vi "Prompt for Step.vi"(0 "Enable":bool=TRUE, 1 "Steps in":T2[](array[typedef]), 3 "Index In":i32=-1, 5 "error in (no error)":errorcluster) -> (16 "New Data Out":T2={"Type"=enum."Mouse Move", "Coords"={"x"=0, "y"=0}, "Delay"=0, "Key"=65, "Repeat"=0, "RClick?"=FALSE}, 18 "OK":bool, 19 "error out":errorcluster)   [LabVIEW 2021]
doc: "Prompts to enter a new step in the profile."
uses:
  CTLs/Step.ctl
  CTLs/Step Type.ctl
  <vilib>/Utility/inputDevices.llb/mouseAcquire.vi
  <vilib>/Utility/inputDevices.llb/closeMouse.vi
panel:
  in  "Repeat Amount":i32 min=0
  in  "Tab Control":enum32{"Coords", "RClick", "Key", "Nothing"}(tab)
  in  "Coords":cluster{"horizontal":i32, "vertical":i32}
  in  "Right Click?":bool
  in  "Key":u8(ring)=65
  in  "Delay (ms)":i32=100 min=0
  out "Step Type Description":string
  in  "Step Type":T1
  in  "Cancel":bool
  in  "OK":bool caption="OK2"
  # "Left and right click at\nsame time to capture\ncurrent screen coords"
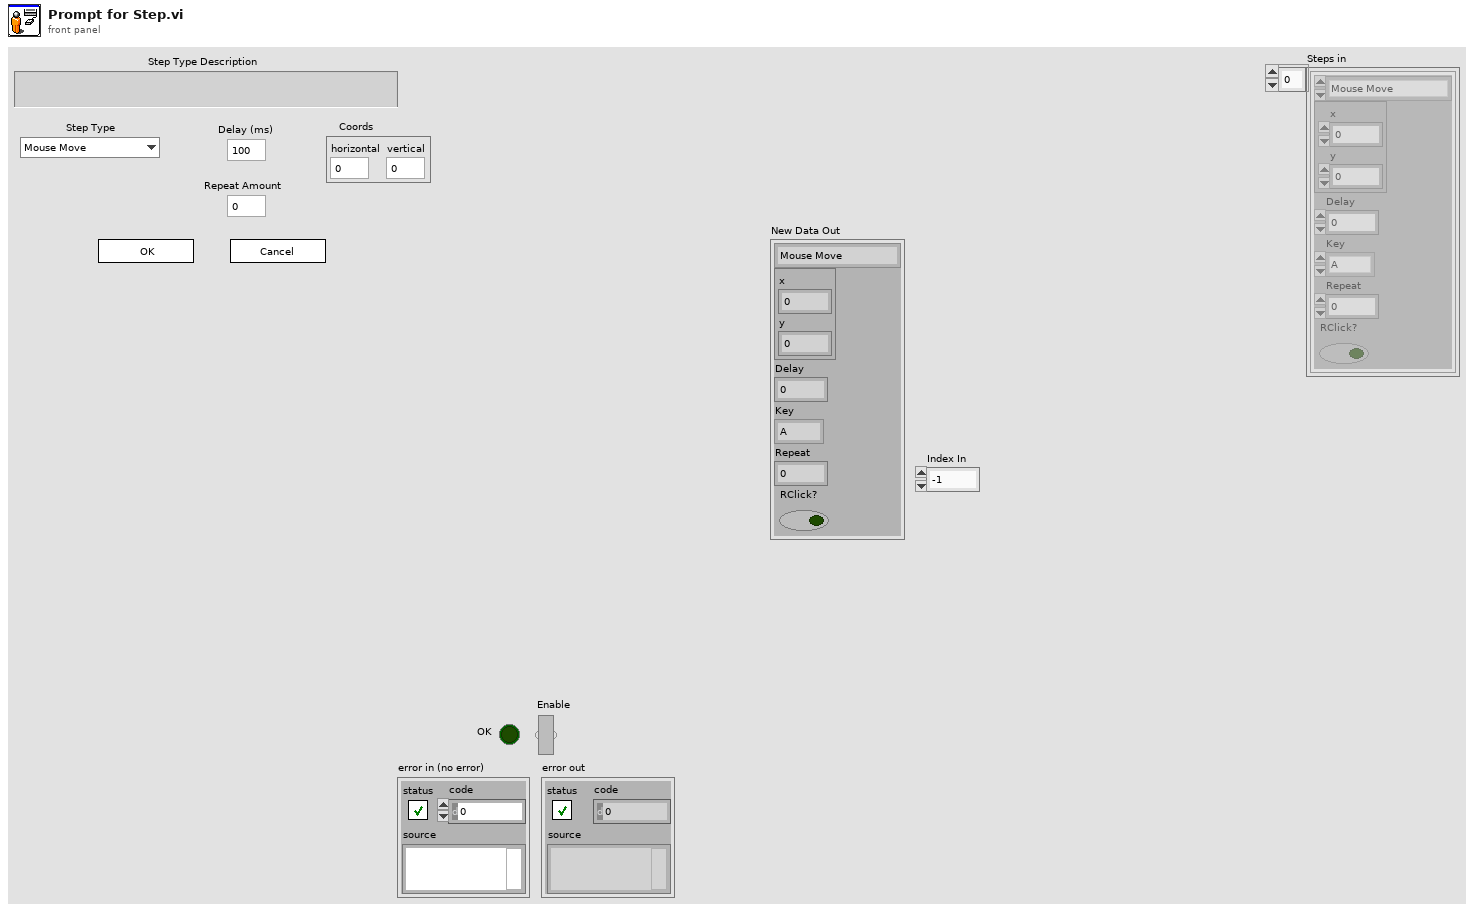
[diagram p1: front panel]
types:
  T1 = typedef "Step Type.ctl" = enum16{"Mouse Move", "Mouse Click", "Key Press", "Wait", "Mouse Down", "Mouse Up", "Key Down", "Key Up"}
  T2 = typedef "Step.ctl" = cluster{"Type":T1, "Coords":cluster{"x":i32, "y":i32}, "Delay":i32, "Key":u8, "Repeat":i32, "RClick?":bool}
  T3 = cluster{"Horizontal":i32, "Vertical":i32, "Scrolling":i32}
  T4 = cluster{"button 1":bool, "button 2":bool, "button 3":bool, "button 4":bool}
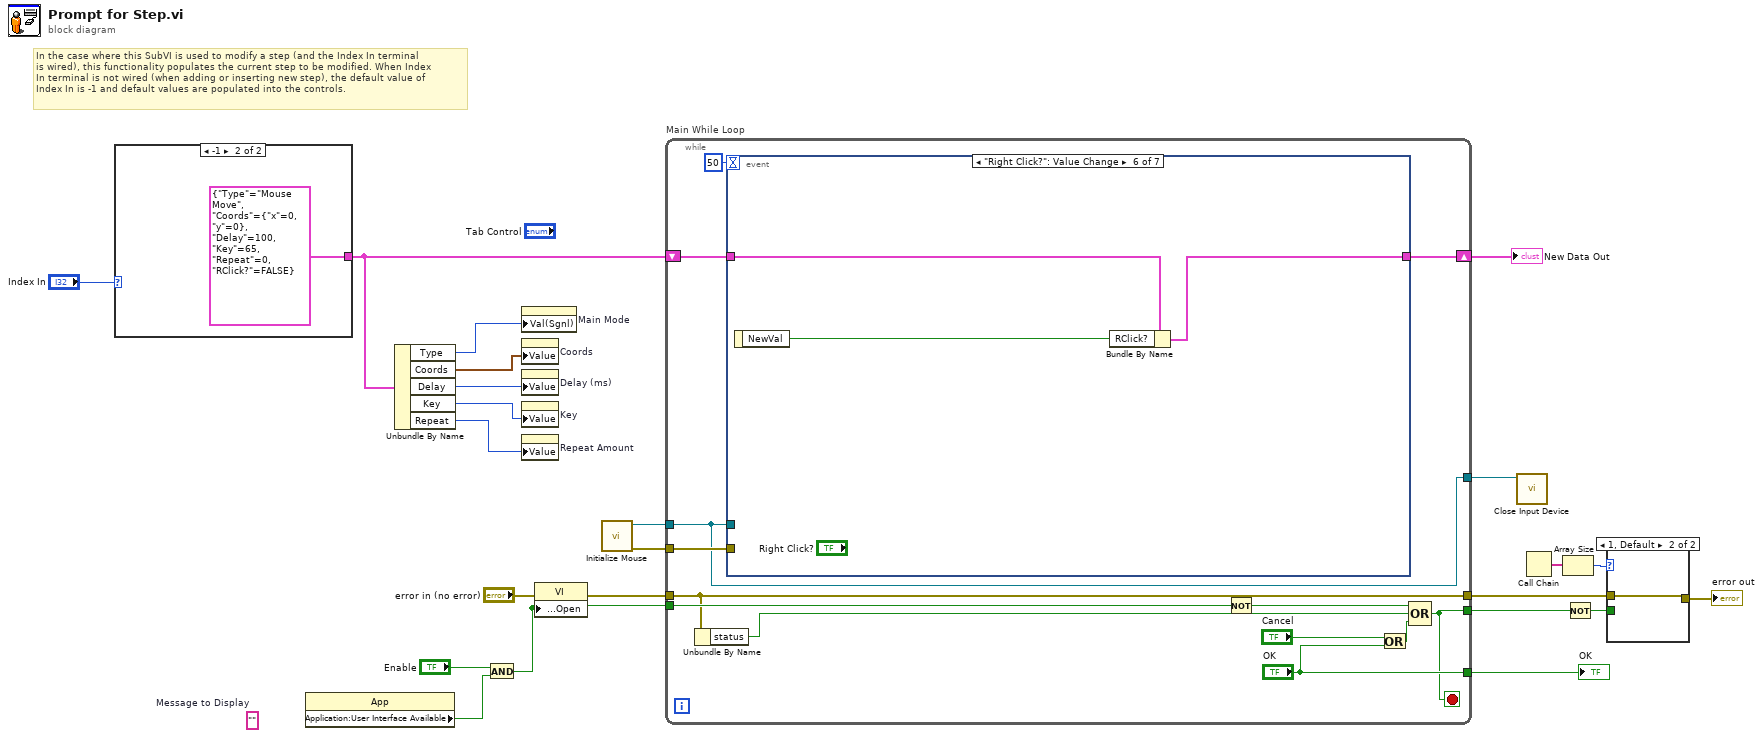
[diagram p0: block diagram]
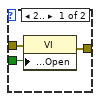
[diagram p2: hidden frame]
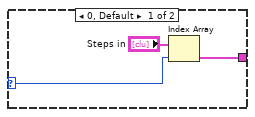
[diagram p3: hidden frame]
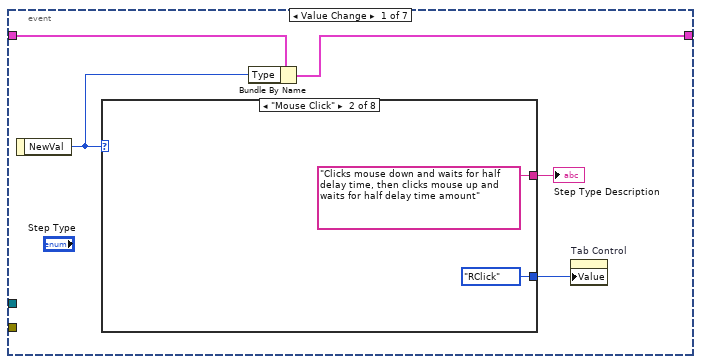
[diagram p4: hidden frame]
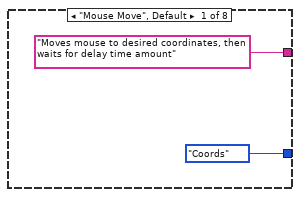
[diagram p5: hidden frame]
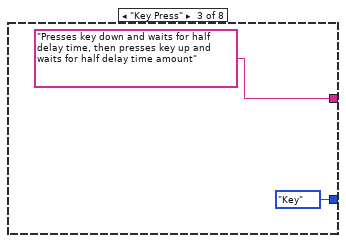
[diagram p6: hidden frame]
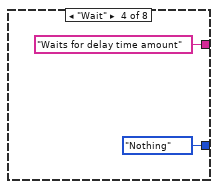
[diagram p7: hidden frame]
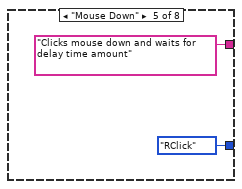
[diagram p8: hidden frame]
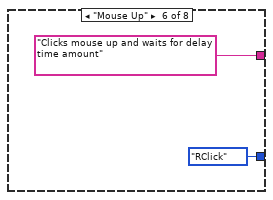
[diagram p9: hidden frame]
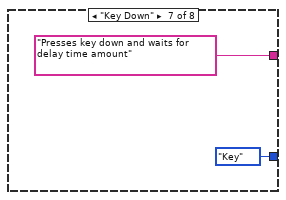
[diagram p10: hidden frame]
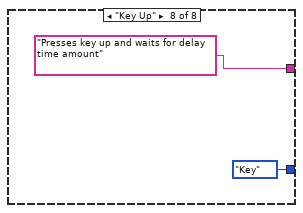
[diagram p11: hidden frame]
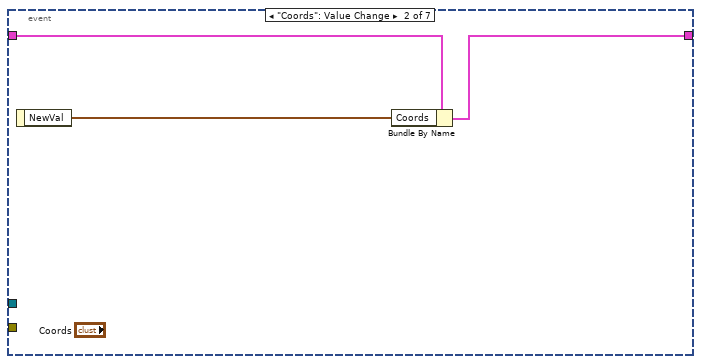
[diagram p12: hidden frame]
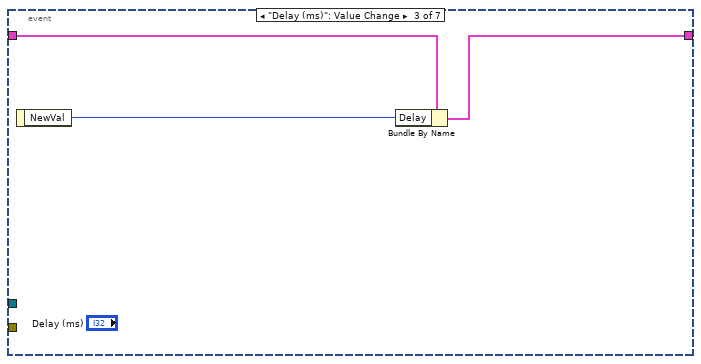
[diagram p13: hidden frame]
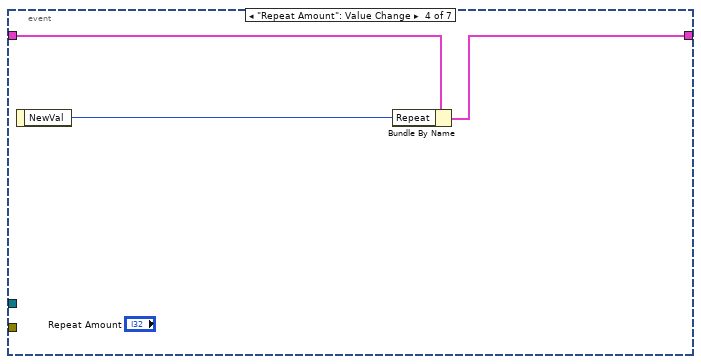
[diagram p14: hidden frame]
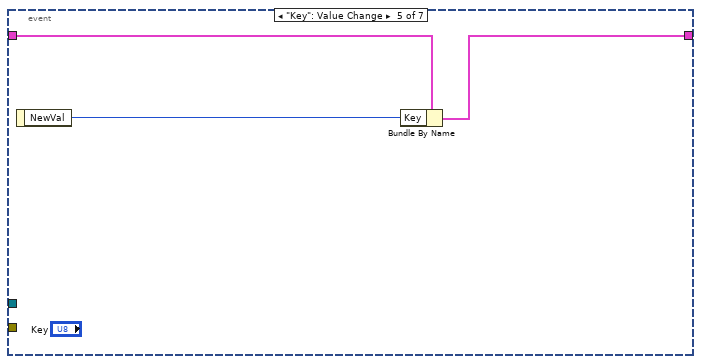
[diagram p15: hidden frame]
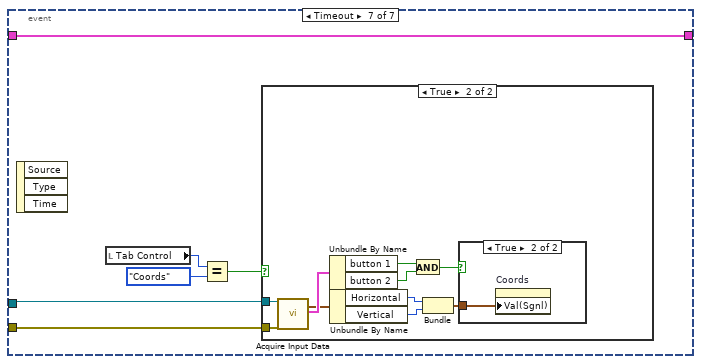
[diagram p16: hidden frame]
diagram:
  (unwired) ""  # Message to Display
  # "In the case where this SubVI is used to modify a step (and the Index In terminal\nis wired), this functionality populates the current step to be modified. When Index\nIn terminal is not wired (when adding or inserting new step), the default value of\nIndex In is -1 and default values are populated into the controls."
  n1 = case shown="-1" "Index In" {
    selector: "Index In" -> [w26 _]
    tunnel: [w24 T2 {"Type"=enum."Mouse Move", "Coords"={"x"=0, "y"=0}, "Delay"=100, "Key"=65, "Repeat"=0, "RClick?"=FALSE} ("Cluster")] -> w10
    frame 0, Default {
      n2 = Index Array(array="Steps in", index=w26) -> (element=w24:T2)
    }
    frame -1 {
    }
  }
  n3 = property class="App"() -> ("Application:User Interface Available"=w15:bool)  [unwired: 2 in, 2 out]
  n4 = Unbundle By Name(w10) -> ("Type"=w11:T1, "Coords"=w9:cluster{"x":i32, "y":i32}, "Delay"=w7:i32, "Key"=w8:u8, "Repeat"=w6:i32)
  n5 = And(x="Enable", y=w15) -> (x .and. y?=w16:bool)
  n6 = property on="Main Mode" class="Enum (strict)"("Val(Sgnl)"=w11) -> ()  [unwired: 2 in, 2 out]
  n7 = property on="Coords" class="Clust (strict)"("Value"=w9) -> ()  [unwired: 2 in, 2 out]
  n8 = property on="Delay (ms)" class="DigNum (strict)"("Value"=w7) -> ()  [unwired: 2 in, 2 out]
  n9 = property on="Key" class="Ring (strict)"("Value"=w8) -> ()  [unwired: 2 in, 2 out]
  n10 = property on="Repeat Amount" class="DigNum (strict)"("Value"=w6) -> ()  [unwired: 2 in, 2 out]
  n11 = property class="VI"(error in="error in (no error)", "Front Panel Window:Open"=w16) -> (error out=w14:errorcluster)  [unwired: 1 in, 1 out]
  n12 = call <vilib>:"Initialize Mouse.vi"() -> ("error out"=w4:errorcluster, "device ID"=w5:refnum<k1>)  [unwired: 10 in]
  n13 = while "Main While Loop" {
    tunnel: ["OK"] -> w23
    tunnel: w16 -> [w38]
    tunnel: [w36] -> w21
    tunnel: w14 -> [w35]
    tunnel: [w35] -> w19
    shift-right: [w31] -> w13
    shift-left: w10 -> [w32]
    tunnel: w4 -> [w29]
    tunnel: w5 -> [w28]
    tunnel: [w28] -> w3
    stop <- w36 stop-if-true
    n14 = Unbundle By Name(w35) -> ("status"=w33:bool)
    n15 = event shown="[5] \"Right Click?\": Value Change" {
      selector: _ -> [_ _ _ _ _ _ _]
      dyn-events: _ -> [_ _ _ _ _ _ _]
      timeout: 50 -> [_ _ _ _ _ _ _]
      tunnel: w32 -> [w43 w64 w67 w70 w73 w76 w82]
      tunnel: [w42 w63 w66 w69 w72 w75 w82] -> w31
      tunnel: w28 -> [_ _ _ _ _ _ w80]
      tunnel: w29 -> [_ _ _ _ _ _ w81]
      event Value Change {
        n16 = event-data() -> ("NewVal"=w41:T1)  [unwired: 1 in]
        n17 = case shown="\"Mouse Click\"" w41 {
          tunnel: ["Moves mouse to desired coordinates, then waits for delay time amount" "Clicks mouse down and waits for half delay time, then clicks mouse up and waits for half delay time amount" "Presses key down and waits for half delay time, then presses key up and waits for half delay time amount" "Waits for delay time amount" "Clicks mouse down and waits for delay time amount" "Clicks mouse up and waits for delay time amount" "Presses key down and waits for delay time amount" "Presses key up and waits for delay time amount"] -> w45
          tunnel: [enum32{"Coords", "RClick", "Key", "Nothing"}."Coords" ("Tab Control") enum32{"Coords", "RClick", "Key", "Nothing"}."RClick" ("Tab Control") enum32{"Coords", "RClick", "Key", "Nothing"}."Key" ("Tab Control") enum32{"Coords", "RClick", "Key", "Nothing"}."Nothing" ("Tab Control") enum32{"Coords", "RClick", "Key", "Nothing"}."RClick" ("Tab Control") enum32{"Coords", "RClick", "Key", "Nothing"}."RClick" ("Tab Control") enum32{"Coords", "RClick", "Key", "Nothing"}."Key" ("Tab Control") enum32{"Coords", "RClick", "Key", "Nothing"}."Key" ("Tab Control")] -> w44
          frame "Mouse Move", Default {
          }
          frame "Mouse Click" {
          }
          frame "Key Press" {
          }
          frame "Wait" {
          }
          frame "Mouse Down" {
          }
          frame "Mouse Up" {
          }
          frame "Key Down" {
          }
          frame "Key Up" {
          }
        }
        "Step Type Description" <- w45
        n18 = Bundle By Name(cluster=w43, "Type"=w41) -> (w42:T2)
        n19 = property on="Tab Control" class="TabCtl (strict)"("Value"=w44) -> ()  [unwired: 2 in, 2 out]
      }
      event "Coords": Value Change {
        n20 = event-data() -> ("NewVal"=w62:cluster{"horizontal":i32, "vertical":i32})  [unwired: 1 in]
        n21 = Bundle By Name(cluster=w64, "Coords"=w62) -> (w63:T2)
      }
      event "Delay (ms)": Value Change {
        n22 = event-data() -> ("NewVal"=w65:i32)  [unwired: 1 in]
        n23 = Bundle By Name(cluster=w67, "Delay"=w65) -> (w66:T2)
      }
      event "Repeat Amount": Value Change {
        n24 = event-data() -> ("NewVal"=w68:i32)  [unwired: 1 in]
        n25 = Bundle By Name(cluster=w70, "Repeat"=w68) -> (w69:T2)
      }
      event "Key": Value Change {
        n26 = event-data() -> ("NewVal"=w71:u8)  [unwired: 1 in]
        n27 = Bundle By Name(cluster=w73, "Key"=w71) -> (w72:T2)
      }
      event "Right Click?": Value Change {
        n28 = event-data() -> ("NewVal"=w74:bool)  [unwired: 1 in]
        n29 = Bundle By Name(cluster=w76, "RClick?"=w74) -> (w75:T2)
      }
      event Timeout {
        n30 = event-data() -> ()  [unwired: 1 in, 3 out]
        n31 = local read "Tab Control"() -> (w79:enum32{"Coords", "RClick", "Key", "Nothing"})
        n32 = Equal?(x=w79, y=enum32{"Coords", "RClick", "Key", "Nothing"}."Coords") -> (x = y?=w77:bool)
        n33 = case shown="True" w77 {
          tunnel: w81 -> [_ w92]
          tunnel: w80 -> [_ w91]
          frame False {
          }
          frame True {
            n34 = call-poly <vilib>:"Acquire Input Data.vi"("device ID"=w91, "error in (no error)"=w92) -> ("axis info"=w89:T3, "button info"=w90:T4)  [unwired: 14 in, 2 out]
            n35 = Unbundle By Name(w90) -> ("button 1"=w84:bool, "button 2"=w85:bool)
            n36 = Unbundle By Name(w89) -> ("Horizontal"=w88:i32, "Vertical"=w87:i32)
            n37 = And(x=w84, y=w85) -> (x .and. y?=w83:bool)
            n38 = Bundle("Horizontal"=w88, "Vertical"=w87) -> (w86:cluster{"Horizontal":i32, "Vertical":i32})  [unwired: 1 in]
            n39 = case shown="True" w83 {
              tunnel: w86 -> [_ w93]
              frame False {
              }
              frame True {
                n40 = property on="Coords" class="Clust (strict)"("Val(Sgnl)"=w93) -> ()  [unwired: 2 in, 2 out]
              }
            }
          }
        }
      }
    }
    n41 = Not(x=w38) -> (.not. x?=w37:bool)
    n42 = Or(x="Cancel", y="OK") -> (x .or. y?=w34:bool)
    n43 = Compound Arithmetic op=OR(w37, w33, w34) -> (w36:bool)
  }
  "OK" <- w23
  "New Data Out" <- w13
  n44 = call-poly <vilib>:"Close Input Device.vi"("device ID"=w3) -> ()  [unwired: 9 in, 1 out]
  n45 = Call Chain() -> (call chain=w2:string[])
  n46 = Array Size(array=w2) -> (size(s)=w1:i32)
  n47 = Not(x=w21) -> (.not. x?=w22:bool)
  n48 = case shown="1, Default" w1 {
    tunnel: w22 -> [w96 _]
    tunnel: w19 -> [w95 w97]
    tunnel: [w94 w97] -> w18
    frame 2.. {
      n49 = property class="VI"(error in=w95, "Front Panel Window:Open"=w96) -> (error out=w94:errorcluster)  [unwired: 1 in, 1 out]
    }
    frame 1, Default {
    }
  }
  "error out" <- w18
